vi "Array Delete Empty.vi"(11 "input":string[](array[string])) -> (3 "output":string[](array[string]))   [LabVIEW 2011]
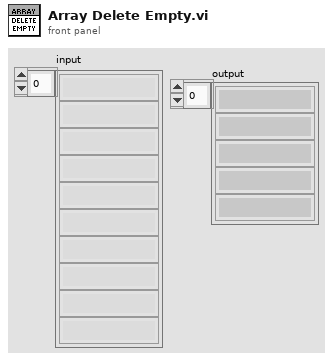
[diagram p1: front panel]
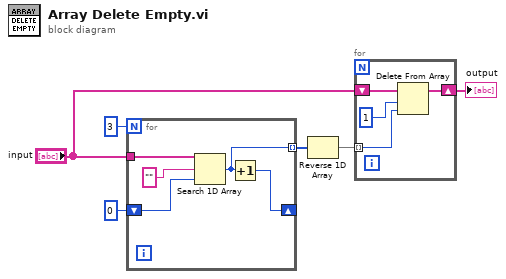
[diagram p0: block diagram]
diagram:
  n1 = for {
    N: 3 -> [_]
    tunnel: "input" -> [w11]
    shift-right: [w10] -> _
    shift-left: 0 ("index of element") -> [w9]
    tunnel: [w7] -> w4 mode=indexing
    n2 = Search 1D Array(1D array=w11, element="" ("元素"), start index (0)=w9) -> (index of element=w7:i32)
    n3 = Increment(x=w7) -> (x+1=w10:i32)
  }
  n4 = Reverse 1D Array(array=w4) -> (reversed array=w3:i32[])
  n5 = for {
    tunnel: w3 -> [w15] mode=indexing
    shift-right: [w13] -> w2
    shift-left: "input" -> [w12]
    n6 = Delete From Array(array=w12, length=1 ("长度"), index=w15) -> (array with subset deleted=w13:string[])  [unwired: 1 out]
  }
  "output" <- w2
